vi "Configure Dialog.vi"(8 "error in (no error)":errorcluster, 11 "Disable All Sparse Markers [SM] Msg in":refnum<class "Disable All Sparse Markers [SM] Msg.lvclass">) -> (0 "error out":errorcluster, 2 "Ok?":bool, 3 "Disable All Sparse Markers [SM] Msg out":refnum<class "Disable All Sparse Markers [SM] Msg.lvclass">)   [LabVIEW 2014, in "CS++Fgen.lvlib" / "Disable All Sparse Markers [SM] Msg.lvclass"]
uses:
  Disable All Sparse Markers [SM] Msg.lvclass
  Disable All Sparse Markers [SM] Msg.lvclass/Disable All Sparse Markers [SM] Msg.ctl
panel:
  in  "Disable?":bool
  in  "OK Button":bool
  in  "Cancel Button":bool
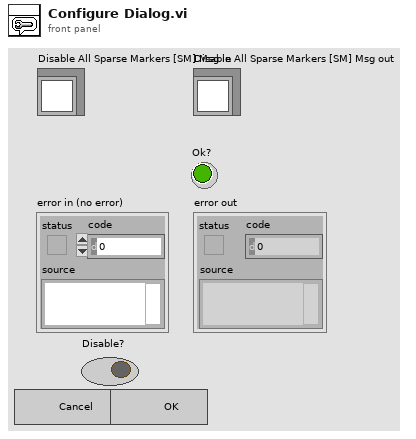
[diagram p1: front panel]
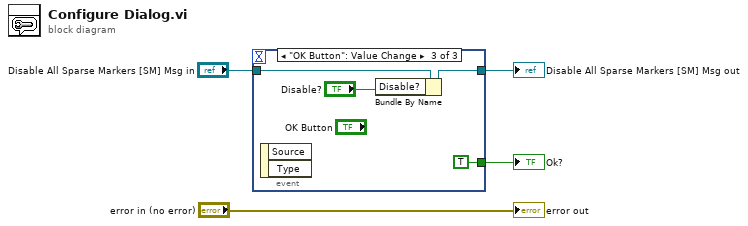
[diagram p0: block diagram]
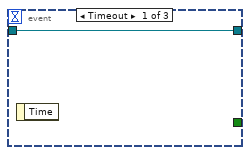
[diagram p2: hidden frame]
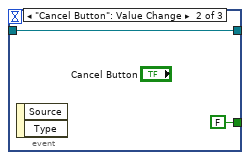
[diagram p3: hidden frame]
diagram:
  n1 = event shown="[2] \"OK Button\": Value Change" {
    selector: _ -> [_ _ _]
    dyn-events: _ -> [_ _ _]
    timeout: _ -> [_ _ _]
    tunnel: [w5 w7 w9] -> w3
    tunnel: "Disable All Sparse Markers [SM] Msg in" -> [w5 w7 w11]
    tunnel: [_ FALSE TRUE] -> w1
    event Timeout {
      n2 = event-data() -> ()  [unwired: 1 in, 1 out]
    }
    event "Cancel Button": Value Change {
      n3 = event-data() -> ()  [unwired: 1 in, 2 out]
    }
    event "OK Button": Value Change {
      n4 = event-data() -> ()  [unwired: 1 in, 2 out]
      n5 = Bundle By Name(cluster=w11, "Disable?"="Disable?") -> (w9:refnum<class "Disable All Sparse Markers [SM] Msg.lvclass">)
    }
  }
  "Disable All Sparse Markers [SM] Msg out" <- w3
  "Ok?" <- w1
  "error out" <- "error in (no error)"
